vi "Output_MI.vi"(0 "Machine Interface Actor in":refnum<class "Machine Interface.lvclass">, 5 "Output Cluster_MI":T1, 7 "State":string, 9 "Sub State":string, 11 "error in (no error)":errorcluster) -> (4 "Machine Interface Actor out":refnum<class "Machine Interface.lvclass">, 15 "error out":errorcluster)   [LabVIEW 2019, in "Machine Interface.lvclass"]
uses:
  Machine Interface.lvclass
  Inspection Statemachine/Inspection Statemachine Messages/Acknowledgement_SM Msg/Acknowledgement_SM.lvclass
  <vilib>/ActorFramework/Actor/Actor.lvclass
  Inspection Statemachine/Inspection Statemachine Messages/HardwareActionAck_SM Msg/HardwareActionAck_SM Msg.lvclass
  Common/Controls/Diagnostics Result.ctl
  Inspection Statemachine/Inspection Statemachine Messages/ErrorMessage_SM Msg/ErrorMessage_SM Msg.lvclass
  Inspection Statemachine/Inspection Statemachine Messages/CallLoadingBar_SM Msg/LoadingBar_SM Msg.lvclass
  Inspection Statemachine/Inspection Statemachine Messages/ButtonPressed_SM Msg/ButtonPressed_SM Msg.lvclass
  Inspection Statemachine/Inspection Statemachine Messages/DiagnosticsResult_SM Msg/DiagnosticsResult_SM Msg.lvclass
  C:/Program Files/National Instruments/LabVIEW 2019/vi.lib/ActorFramework/Actor/Actor.lvclass
  <vilib>/ActorFramework/Message Enqueuer/Message Enqueuer.lvclass
  Common/Controls/Acknowledgement.ctl
  Controls/Output Cluster_MI.ctl
  Common/Controls/Pop-up Input.ctl
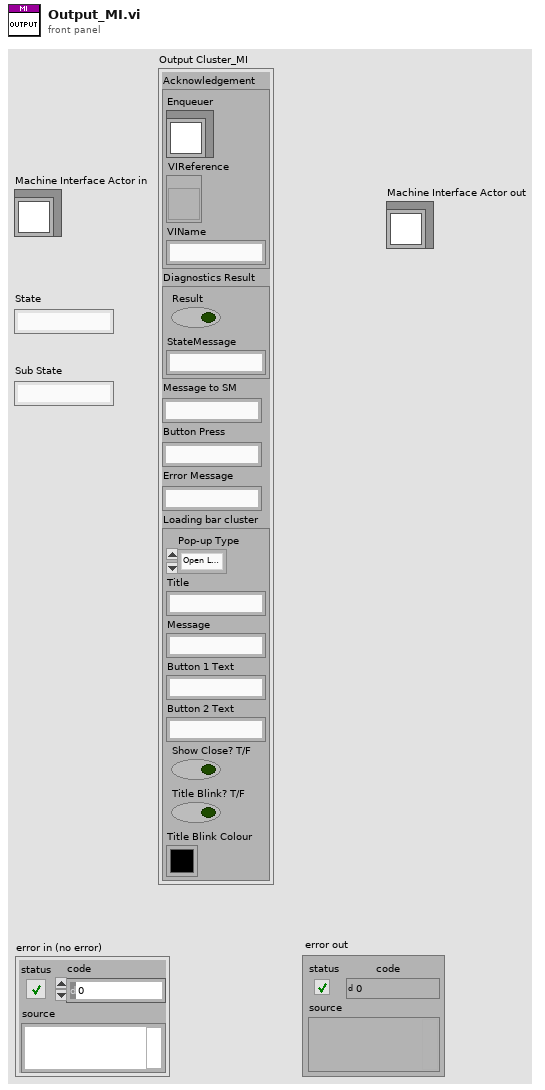
[diagram p1: front panel]
types:
  T1 = typedef "Machine Interface.lvclass/Output Cluster_MI.ctl" = cluster{"Acknowledgement":T2, "Diagnostics Result":T3, "Message to SM":string, "Button Press":string, "Error Message":string, "Loading bar cluster":T4}
  T2 = typedef "Acknowledgement.ctl" = cluster{"Enqueuer":refnum<class "Message Enqueuer.lvclass">, "VIReference":refnum<vi>, "VIName":string}
  T3 = typedef "Diagnostics Result.ctl" = cluster{"Result":bool, "StateMessage":string}
  T4 = typedef "Pop-up Input.ctl" = cluster{"Pop-up Type":enum16{"Open Logo Display", "Close Logo Display", "Open Loading Bar", "Close Loading Bar", "Open Alert Display", "Close Alert Display", "One button dialog box", "Two button dialog box", "User Authentication"}, "Title":string, "Message":string, "Button 1 Text":string, "Button 2 Text":string, "Show Close? T/F":bool, "Title Blink? T/F":bool, "Title Blink Colour":u32}
  T5 = enum16{"Open Logo Display", "Close Logo Display", "Open Loading Bar", "Close Loading Bar", "Open Alert Display", "Close Alert Display", "One button dialog box", "Two button dialog box", "User Authentication"}
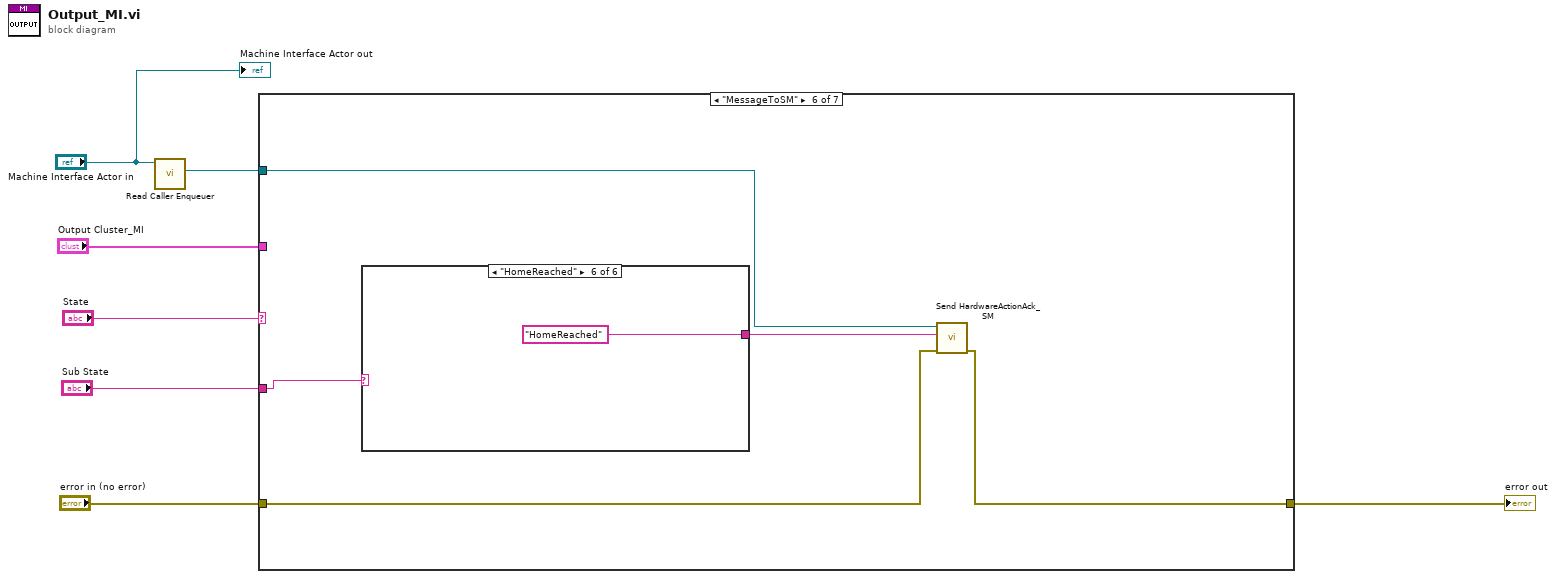
[diagram p0: block diagram]
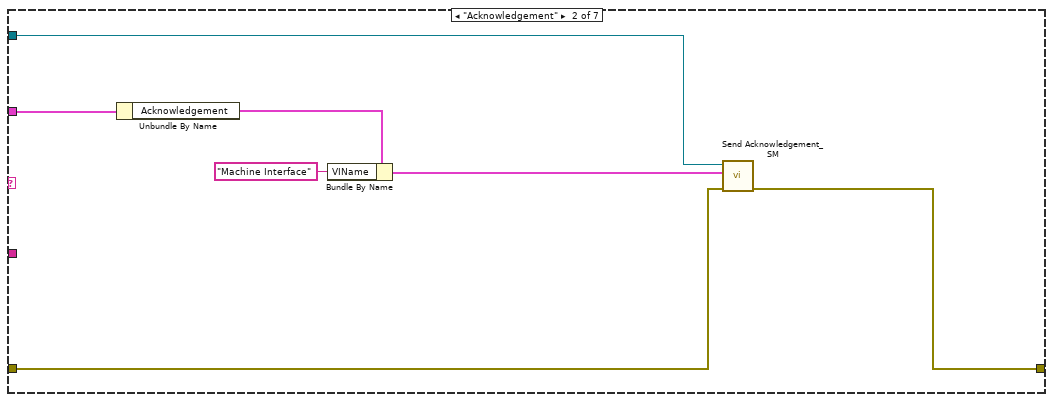
[diagram p3: hidden frame]
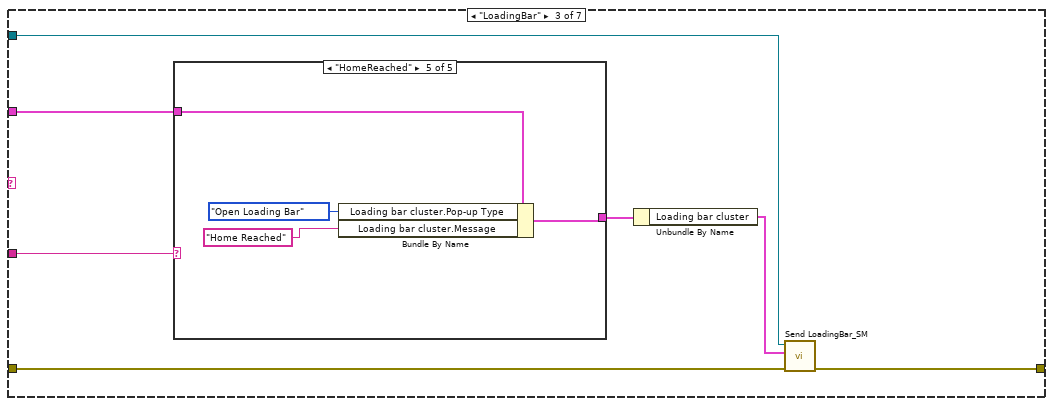
[diagram p4: hidden frame]
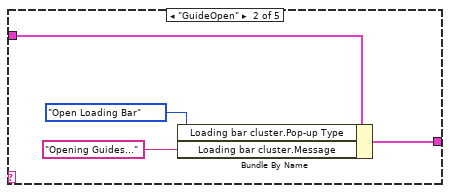
[diagram p6: hidden frame]
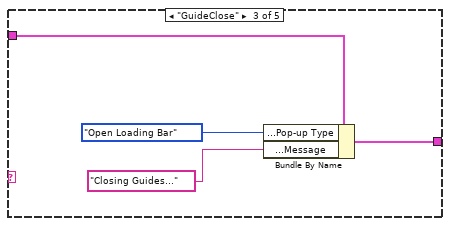
[diagram p7: hidden frame]
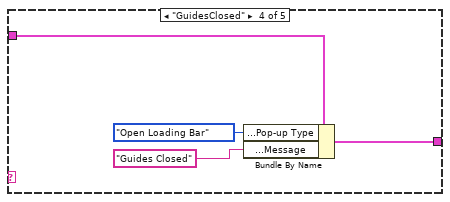
[diagram p8: hidden frame]
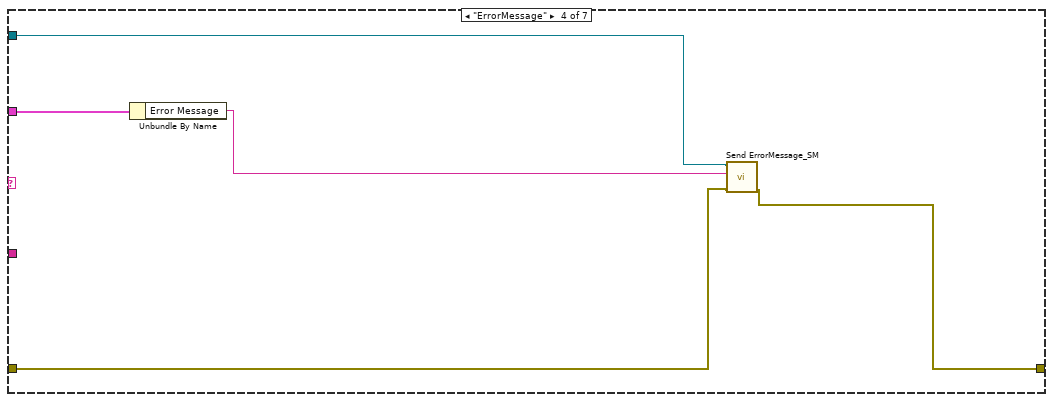
[diagram p9: hidden frame]
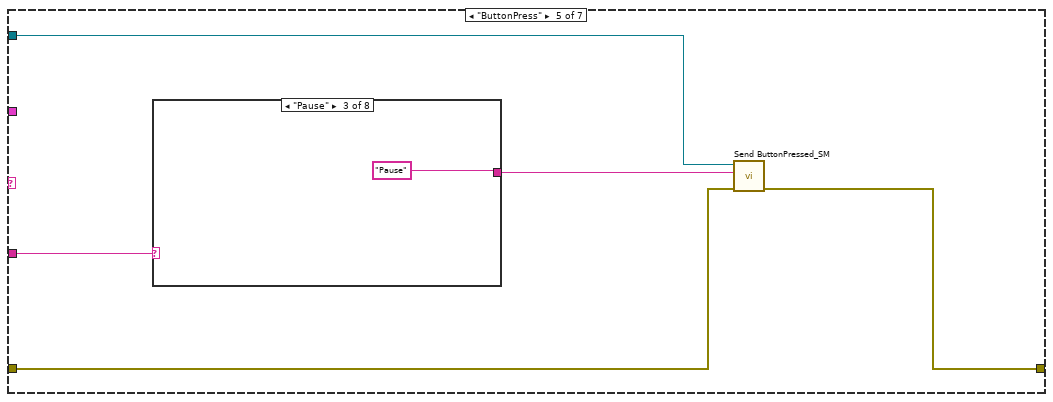
[diagram p10: hidden frame]
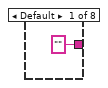
[diagram p11: hidden frame]
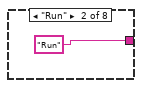
[diagram p12: hidden frame]
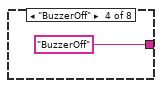
[diagram p13: hidden frame]
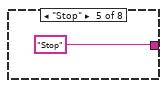
[diagram p14: hidden frame]
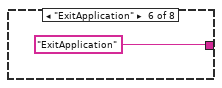
[diagram p15: hidden frame]
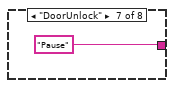
[diagram p16: hidden frame]
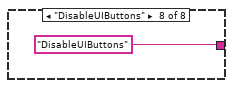
[diagram p17: hidden frame]
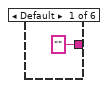
[diagram p18: hidden frame]
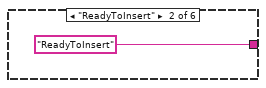
[diagram p19: hidden frame]
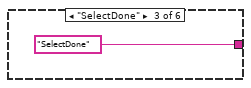
[diagram p20: hidden frame]
diagram:
  n1 = call <vilib>:"Read Caller Enqueuer.vi"("Actor"="Machine Interface Actor in") -> ("Caller Enqueuer"=w3:refnum<class "Message Enqueuer.lvclass">)  [unwired: 10 in]
  n2 = case shown="\"MessageToSM\"" "State" {
    tunnel: "Output Cluster_MI" -> [_ w12 w18 w44 _ _ w75]
    tunnel: w3 -> [_ w13 w20 w41 w46 w61 w72]
    tunnel: "error in (no error)" -> [w8 w15 w22 w43 w48 w59 w71]
    tunnel: [w8 w14 w21 w42 w47 w58 w70] -> w4
    tunnel: "Sub State" -> [_ _ w19 _ w49 w62 w74]
    frame Default {
    }
    frame "Acknowledgement" {
      n3 = Unbundle By Name(w12) -> ("Acknowledgement"=w11:T2)
      n4 = Bundle By Name(cluster=w11, "VIName"="Machine Interface" ("VI Name")) -> (w9:T2)
      n5 = call "Send Acknowledgement_SM.vi"("error in (no error)"=w15, "Acknowledgement"=w9, "Message Enqueuer"=w13) -> ("error out"=w14:errorcluster)  [unwired: 7 in, 1 out]
    }
    frame "LoadingBar" {
      n6 = case shown="\"HomeReached\"" w19 {
        tunnel: [w23 w26 w30 w34 w37] -> w16
        tunnel: w18 -> [w23 w25 w29 w33 w38]
        frame Default {
        }
        frame "GuideOpen" {
          n7 = Bundle By Name(cluster=w25, "Loading bar cluster.Pop-up Type"=T5."Open Loading Bar", "Loading bar cluster.Message"="Opening Guides..." ("event data")) -> (w26:T1)
        }
        frame "GuideClose" {
          n8 = Bundle By Name(cluster=w29, "Loading bar cluster.Pop-up Type"=T5."Open Loading Bar", "Loading bar cluster.Message"="Closing Guides..." ("event data")) -> (w30:T1)
        }
        frame "GuidesClosed" {
          n9 = Bundle By Name(cluster=w33, "Loading bar cluster.Pop-up Type"=T5."Open Loading Bar", "Loading bar cluster.Message"="Guides Closed" ("event data")) -> (w34:T1)
        }
        frame "HomeReached" {
          n10 = Bundle By Name(cluster=w38, "Loading bar cluster.Pop-up Type"=T5."Open Loading Bar", "Loading bar cluster.Message"="Home Reached" ("event data")) -> (w37:T1)
        }
      }
      n11 = Unbundle By Name(w16) -> ("Loading bar cluster"=w17:T4)
      n12 = call "Send LoadingBar_SM.vi"("error in (no error)"=w22, "Pop-up"=w17, "Message Enqueuer"=w20) -> ("error out"=w21:errorcluster)  [unwired: 7 in, 1 out]
    }
    frame "ErrorMessage" {
      n13 = Unbundle By Name(w44) -> ("Error Message"=w40:string)
      n14 = call "Send ErrorMessage_SM.vi"("error in (no error)"=w43, "Error Message"=w40, "Message Enqueuer"=w41) -> ("error out"=w42:errorcluster)  [unwired: 7 in, 1 out]
    }
    frame "ButtonPress" {
      n15 = case shown="\"Pause\"" w49 {
        tunnel: ["" ("Button Press") "Run" ("Button Press") "Pause" ("Button Press") "BuzzerOff" ("Button Press") "Stop" ("Button Press") "ExitApplication" ("Button Press") "Pause" ("Button Press") "DisableUIButtons" ("Button Press")] -> w45
        frame Default {
        }
        frame "Run" {
        }
        frame "Pause" {
        }
        frame "BuzzerOff" {
        }
        frame "Stop" {
        }
        frame "ExitApplication" {
        }
        frame "DoorUnlock" {
        }
        frame "DisableUIButtons" {
        }
      }
      n16 = call "Send ButtonPressed_SM.vi"("error in (no error)"=w48, "ButtonPress"=w45, "Message Enqueuer"=w46) -> ("error out"=w47:errorcluster)  [unwired: 7 in, 1 out]
    }
    frame "MessageToSM" {
      n17 = case shown="\"HomeReached\"" w62 {
        tunnel: ["" ("Sub State") "ReadyToInsert" ("Sub State") "SelectDone" ("Sub State") "RunPositionReached" ("Sub State") "ReadyToRun" ("Sub State") "HomeReached" ("Sub State")] -> w60
        frame Default {
        }
        frame "ReadyToInsert" {
        }
        frame "SelectDone" {
        }
        frame "RunPositionReached" {
        }
        frame "ReadyToRun" {
        }
        frame "HomeReached" {
        }
      }
      n18 = call "Send HardwareActionAck_SM.vi"("error in (no error)"=w59, "HardwareActionAck"=w60, "Message Enqueuer"=w61) -> ("error out"=w58:errorcluster)  [unwired: 7 in, 1 out]
    }
    frame "DiagnosticsResult" {
      n19 = Unbundle By Name(w75) -> ("Diagnostics Result"=w73:T3)
      n20 = case shown="\"DoorLocked\"" w74 {
        tunnel: w73 -> [_ w78 w82 w86 w91 w94 w98 w102 w106 w110 w116 w120]
        tunnel: [T3 {"Result"=TRUE, "StateMessage"=""} ("Diagnostics Result") w77 w81 w85 w90 w93 w97 w101 w105 w109 w115 w119] -> w69
        frame Default {
        }
        frame "DeviceNotReady" {
          n21 = Bundle By Name(cluster=w78, "Result"=FALSE, "StateMessage"="DeviceNotReady_0x03000101") -> (w77:T3)
        }
        frame "DeviceReady" {
          n22 = Bundle By Name(cluster=w82, "Result"=TRUE, "StateMessage"="DeviceReady") -> (w81:T3)
        }
        frame "MachinePoweredOn" {
          n23 = Bundle By Name(cluster=w86, "Result"=TRUE, "StateMessage"="MachinePoweredOn") -> (w85:T3)
        }
        frame "MachineNotPoweredON" {
          n24 = Bundle By Name(cluster=w91, "Result"=FALSE, "StateMessage"="MachineNotPoweredON_0x03000501") -> (w90:T3)
        }
        frame "MotorDiagnosticsDone" {
          n25 = Bundle By Name(cluster=w94, "Result"=TRUE, "StateMessage"="MotorDiagnosticsDone") -> (w93:T3)
        }
        frame "GuideOpenFail" {
          n26 = Bundle By Name(cluster=w98, "Result"=FALSE, "StateMessage"="MotorDiagnosticsFailed_0x03000200") -> (w97:T3)
        }
        frame "GuideCloseFail" {
          n27 = Bundle By Name(cluster=w102, "Result"=FALSE, "StateMessage"="MotorDiagnosticsFailed_0x03000300") -> (w101:T3)
        }
        frame "ComPortAvailable" {
          n28 = Bundle By Name(cluster=w106, "Result"=TRUE, "StateMessage"="ComPortAvailable") -> (w105:T3)
        }
        frame "ComPortNotAvailable" {
          n29 = Bundle By Name(cluster=w110, "Result"=FALSE, "StateMessage"="ComPortNotAvailable_0x03000100") -> (w109:T3)
        }
        frame "DoorLocked" {
          n30 = Bundle By Name(cluster=w116, "Result"=TRUE, "StateMessage"="DoorLocked") -> (w115:T3)
        }
        frame "DoorUnlocked" {
          n31 = Bundle By Name(cluster=w120, "Result"=FALSE, "StateMessage"="DoorNotLocked") -> (w119:T3)
        }
      }
      n32 = call "Send DiagnosticsResult_SM.vi"("error in (no error)"=w71, "DiagnosticsResult"=w69, "Message Enqueuer"=w72) -> ("error out"=w70:errorcluster)  [unwired: 7 in, 1 out]
    }
  }
  "error out" <- w4
  "Machine Interface Actor out" <- "Machine Interface Actor in"
